vi "CallUserScripting.vi"(8 "error in":errorcluster, 11 "BaseAccessorScripter in":refnum<class "BaseAccessorScripter.lvclass">) -> (0 "error out":errorcluster, 3 "BaseAccessorScripter out":refnum<class "BaseAccessorScripter.lvclass">)   [LabVIEW 2021, in "MemberVICreation.lvlib" / "BaseAccessorScripter.lvclass"]
doc: "This VI provides an opportunity for users to add scripting code of their own to modify the scripting process even if they do not have the password to the VIs in the scripting. Each overriding class should call out to an empty subVI, one that is not a member of the class, that users can edit to put in their own scripting behavior."
uses:
  <resource>/Framework/Providers/LVClassLibrary/NewAccessors/BaseAccessorScripter/BaseAccessorScripter.lvclass
  <resource>/Framework/Providers/LVClassLibrary/NewAccessors/BaseAccessorScripter/BaseAccessorScripter.lvclass/BaseAccessorScripter.ctl
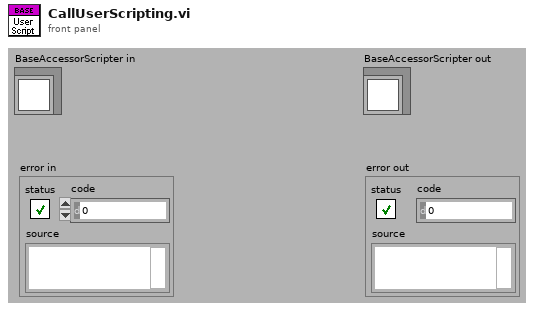
[diagram p1: front panel]
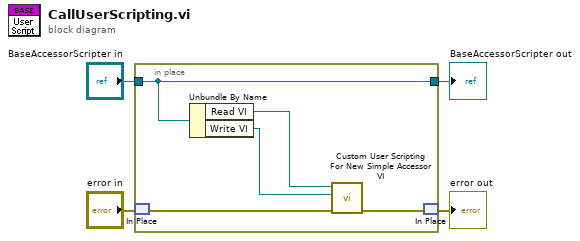
[diagram p0: block diagram]
diagram:
  n1 = in-place {
    in-place-border: [w9] -> w3
    in-place-border: "BaseAccessorScripter in" -> [w9]
    n2 = in-place-match #1("error in") -> (w7:errorcluster)
    n3 = Unbundle By Name(w9) -> ("Read VI"=w6:refnum<vi>, "Write VI"=w5:refnum<vi>)
    n4 = call <resource>:"Custom User Scripting For New Simple Accessor VI.vi"("error in"=w7, "Write VI"=w5, "Read VI"=w6) -> ("error out"=w8:errorcluster)  [unwired: 8 in]
    n5 = in-place-match #1(w8) -> (→"error out":errorcluster)
  }
  "BaseAccessorScripter out" <- w3
